vi "Post-Install Custom Action.vi"(10 "Variant":variant) -> (0 "error out":errorcluster)   [LabVIEW 2017]
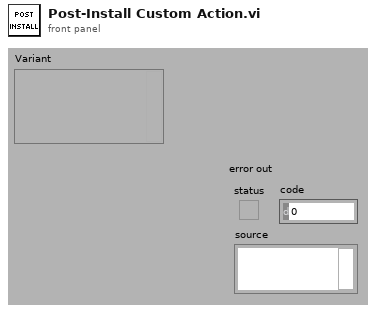
[diagram p1: front panel]
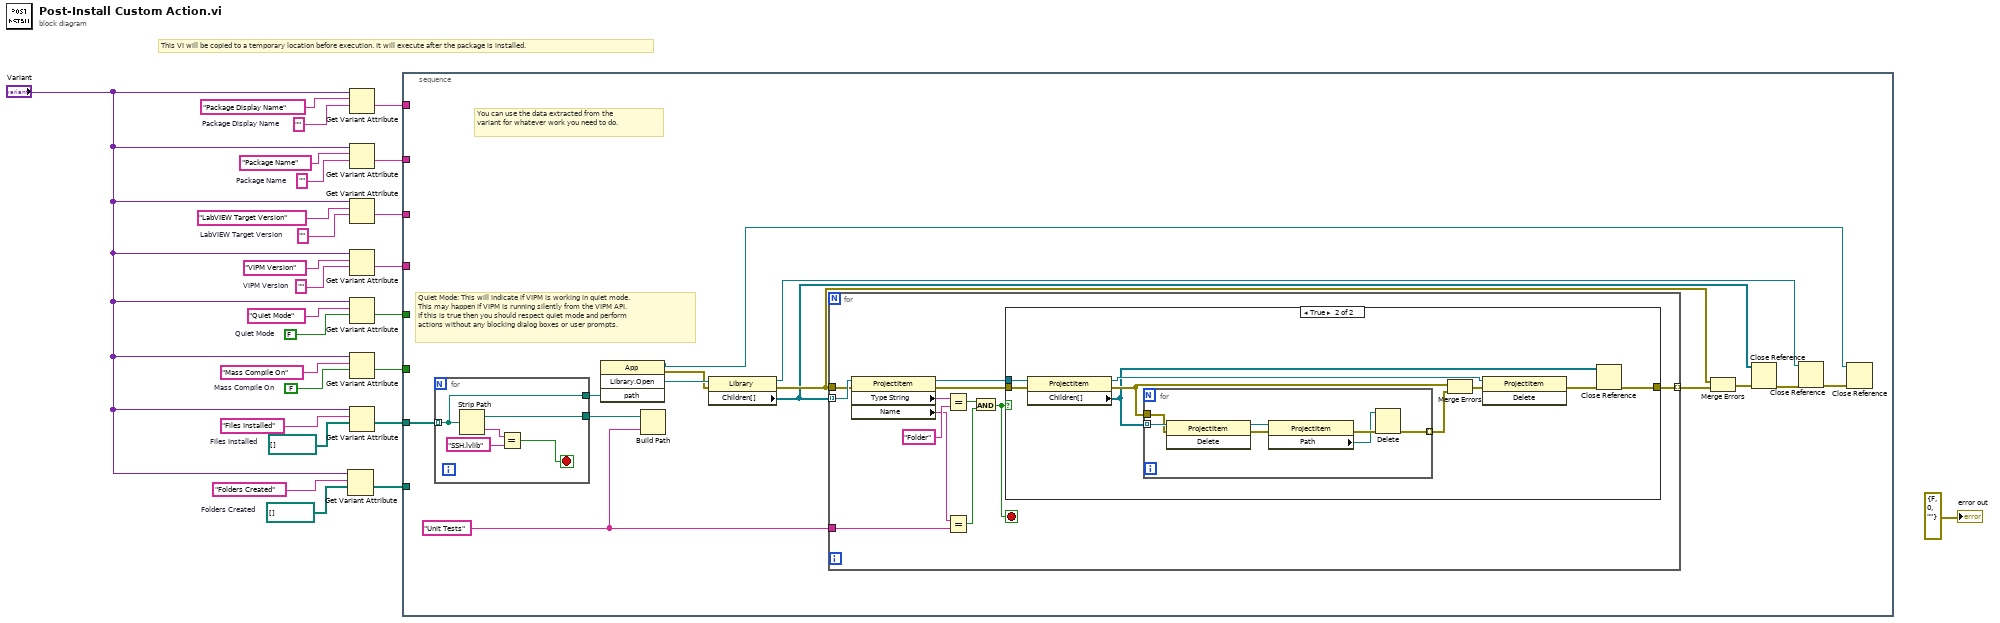
[diagram p0: block diagram]
diagram:
  w1 = path[] []  # Folders Created
  w2 = path[] []  # Files Installed
  w8 = FALSE  # Mass Compile On
  w9 = ""  # Package Display Name
  w16 = FALSE  # Quiet Mode
  w19 = ""  # VIPM Version
  w21 = ""  # LabVIEW Target Version
  w23 = ""  # Package Name
  # "This VI will be copied to a temporary location before execution. It will execute after the package is installed."
  n1 = Get Variant Attribute(Variant="Variant", name="Folders Created", default value (empty Variant)=w1) -> (value=w6:path[])  [unwired: 1 in, 3 out]
  n2 = Get Variant Attribute(Variant="Variant", name="Package Display Name", default value (empty Variant)=w9) -> (value=w15:string)  [unwired: 1 in, 3 out]
  n3 = Get Variant Attribute(Variant="Variant", name="Package Name", default value (empty Variant)=w23) -> (value=w14:string)  [unwired: 1 in, 3 out]
  n4 = Get Variant Attribute(Variant="Variant", name="LabVIEW Target Version", default value (empty Variant)=w21) -> (value=w13:string)  [unwired: 1 in, 3 out]
  n5 = Get Variant Attribute(Variant="Variant", name="VIPM Version", default value (empty Variant)=w19) -> (value=w12:string)  [unwired: 1 in, 3 out]
  n6 = Get Variant Attribute(Variant="Variant", name="Quiet Mode", default value (empty Variant)=w16) -> (value=w11:bool)  [unwired: 1 in, 3 out]
  n7 = Get Variant Attribute(Variant="Variant", name="Mass Compile On", default value (empty Variant)=w8) -> (value=w10:bool)  [unwired: 1 in, 3 out]
  n8 = Get Variant Attribute(Variant="Variant", name="Files Installed", default value (empty Variant)=w2) -> (value=w5:path[])  [unwired: 1 in, 3 out]
  n9 = stacked-sequence {
    tunnel: w15 -> [_]
    tunnel: w14 -> [_]
    tunnel: w13 -> [_]
    tunnel: w12 -> [_]
    tunnel: w11 -> [_]
    tunnel: w10 -> [_]
    tunnel: w5 -> [w40]
    tunnel: w6 -> [_]
    frame #0 {
      w36 = "Unit Tests" ("name or relative path")
      # "Quiet Mode: This will indicate if VIPM is working in quiet mode.\nThis may happen if VIPM is running silently from the VIPM API.\nIf this is true then you should respect quiet mode and perform\nactions without any blocking dialog boxes or user prompts."
      # "You can use the data extracted from the variant for whatever work you need to do."
      n10 = for {
        tunnel: w40 -> [w71] mode=indexing
        tunnel: [w71] -> w39
        tunnel: [w70] -> w38
        stop <- w72 stop-if-true
        n11 = Strip Path(path=w71) -> (stripped path=w70:path, name=w74:string)
        n12 = Equal?(x=w74, y="SSH.lvlib") -> (x = y?=w72:bool)
      }
      n13 = invoke class="App" method="Library.Open"("path"=w39) -> (reference out=w27:refnum<vi>, error out=w35:errorcluster, "Open Library"=w37:refnum<vi>)  [unwired: 3 in, 1 out]
      n14 = Build Path(base path=w38, name or relative path=w36) -> ()  [unwired: 1 out]
      n15 = property class="Library"(reference=w37, error in=w35) -> (reference out=w29:refnum<vi>, error out=w32:errorcluster, "Children[]"=w31:refnum<vi>[])
      n16 = for {
        tunnel: w31 -> [w52] mode=indexing
        tunnel: w32 -> [w51]
        tunnel: [w41] -> w33 mode=indexing
        tunnel: w36 -> [w47]
        stop <- w42 stop-if-true
        n17 = property class="ProjectItem"(reference=w52, error in=w51) -> (reference out=w44:refnum<vi>, error out=w43:errorcluster, "Type String"=w50:string, "Name"=w48:string)
        n18 = Equal?(x=w50, y="Folder" ("Type String")) -> (x = y?=w45:bool)
        n19 = Equal?(x=w48, y=w47) -> (x = y?=w46:bool)
        n20 = And(x=w45, y=w46) -> (x .and. y?=w42:bool)
        n21 = case shown="True" w42 {
          tunnel: w44 -> [_ w62]
          tunnel: w43 -> [w53 w61]
          tunnel: [w53 w55] -> w41
          frame False {
          }
          frame True {
            n22 = property class="ProjectItem"(reference=w62, error in=w61) -> (reference out=w56:refnum<vi>, error out=w59:errorcluster, "Children[]"=w54:refnum<vi>[])
            n23 = for {
              tunnel: w54 -> [w69] mode=indexing
              tunnel: w59 -> [w68]
              tunnel: [w64] -> w60 mode=indexing
              n24 = invoke class="ProjectItem" method="Delete"(reference=w69, error in=w68) -> (reference out=w65:refnum<vi>, error out=w67:errorcluster)  [unwired: 1 in, 1 out]
              n25 = property class="ProjectItem"(reference=w65, error in=w67) -> (error out=w66:errorcluster, "Path"=w63:path)  [unwired: 1 out]
              n26 = Delete(path (use dialog)=w63, error in=w66) -> (error out=w64:errorcluster)  [unwired: 3 in, 2 out]
            }
            n27 = Merge Errors(w59, w60) -> (w58:errorcluster)
            n28 = invoke class="ProjectItem" method="Delete"(reference=w56, error in=w58) -> (error out=w57:errorcluster)  [unwired: 1 in, 2 out]
            n29 = Close Reference(reference=w54, error in (no error)=w57) -> (error out=w55:errorcluster)
          }
        }
      }
      n30 = Merge Errors(w32, w33) -> (w34:errorcluster)
      n31 = Close Reference(reference=w31, error in (no error)=w34) -> (error out=w30:errorcluster)
      n32 = Close Reference(reference=w29, error in (no error)=w30) -> (error out=w28:errorcluster)
      n33 = Close Reference(reference=w27, error in (no error)=w28) -> ()  [unwired: 1 out]
    }
  }
  "error out" <- errorcluster {"status"=FALSE, "code"=0, "source"=""} ("error out")
